vi "convert_DVR-to-StringArray.vi"(5 "Delete DVR? (T)":bool=TRUE, 7 "error in (no error)":errorcluster, 8 "multipart message DVR in":refnum<data-value>) -> (1 "error out":errorcluster, 2 "parts":string[](array[string]))   [LabVIEW 2019, in "zmq_multipart_lib.lvlib" / "zmq_multipart_lib.lvclass"]
uses:
  zmq_multipart_lib.lvclass
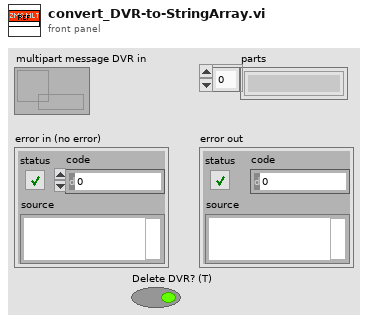
[diagram p1: front panel]
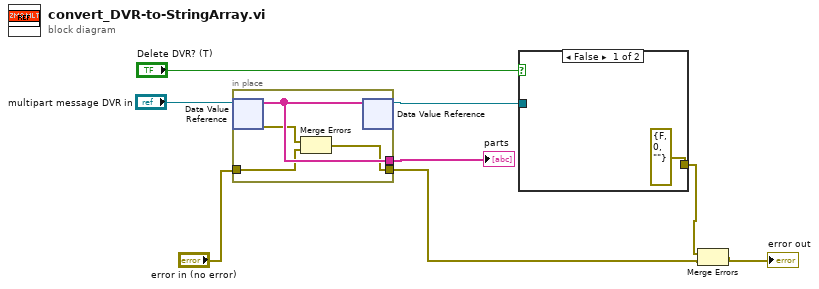
[diagram p0: block diagram]
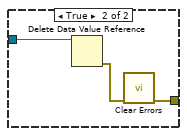
[diagram p2: hidden frame]
diagram:
  n1 = in-place {
    in-place-border: [w12] -> w7
    in-place-border: "error in (no error)" -> [w10]
    in-place-border: [w9] -> w3
    n2 = in-place-dvr #1("multipart message DVR in") -> (w12:string[], w11:errorcluster)
    n3 = Merge Errors(w11, w10) -> (w9:errorcluster)
    n4 = in-place-dvr #1(w12) -> (w5:refnum<data-value>)  [unwired: 1 out]
  }
  "parts" <- w7
  n5 = case shown="False" "Delete DVR? (T)" {
    tunnel: w5 -> [_ w16]
    tunnel: [errorcluster {"status"=FALSE, "code"=0, "source"=""} ("error out") w14] -> w2
    frame False {
    }
    frame True {
      n6 = Delete Data Value Reference(data value reference=w16) -> (error out=w15:errorcluster)  [unwired: 1 in, 1 out]
      n7 = call <vilib>:"Clear Errors.vi"("error in (no error)"=w15) -> ("error out"=w14:errorcluster)  [unwired: 5 in, 1 out]
    }
  }
  n8 = Merge Errors(w2, w3) -> (→"error out":errorcluster)
